vi "3.0-Open FPGA ref and Startup.vi"() -> (0 "queue out":refnum<queue>)   [LabVIEW 2010]
uses:
  2-Low Neurons/2-FPGA VI Typedef.ctl
  2-Low Neurons/2.1-Act Command Typedef.ctl
  2-Low Neurons/2.1 PID Gains Typedef.ctl
  <vilib>/userDefined/High Color/nirio_resource_hc.ctl
  <vilib>/rvi/interface/nirviOpenFPGA/nirviOpenFPGA.xnode
  FPGA Bitfiles/1Hindbrain.lvbitx
  1-Hindbrain.vi
  <vilib>/rvi/ClientSDK/nirviWhatTheDeviceIsDoing.ctl
  <vilib>/rvi/interface/nirviReadWriteControl/nirviReadWriteControl.xnode
  <vilib>/rvi/interface/common/niFpgaNodeNameForErrorReporting.ctl
  <vilib>/rvi/errors/niLvFpgaWhatHappensToTopLevelVI.ctl
  <vilib>/FPGAPlugInAG/cRIO-9104/niLvFpga_Open_cRIO-9104.vi
  <vilib>/Utility/error.llb/Error Cluster From Error Code.vi
  <vilib>/rvi/errors/niLvFpgaAdjustHostInterfaceError.vi
  NiFpgaLv.dll
panel:
  out "error out":errorcluster
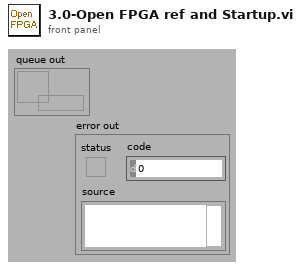
[diagram p1: front panel]
types:
  T1 = typedef "2.1-Act Command Typedef.ctl" = cluster{"Inhibit All Motors":bool, "2.1 Direct Override":bool, "Drive Speed Integer Setpoint":i32, "Steering Integer Setpoint":i32, "Lidar Position Integer Setpoint":i32, "Drive Direct":fxp<+/-,20,5>, "Steer Direct":fxp<+/-,20,5>, "Lidar Direct ":fxp<+/-,20,5>, "2.1.3 Drive PID Gains":T2, "Drive Limit":fxp<+/-,20,5>, "2.1.2 Steering Input C":fxp<+,8,-2>, "2.1.2 Steering Input K":fxp<+/-,14,-6>, "2.1.2 Steering Input F":fxp<+/-,20,5>, "Use NI-9505":bool}
  T2 = typedef "2.1 PID Gains Typedef.ctl" = cluster{"P Gain":fxp<+/-,18,1>, "I Gain":fxp<+/-,18,1>, "D Gain":fxp<+/-,18,1>, "P Gain - Exp":i8, "I Gain - Exp":i8, "D Gain - Exp":i8, "I Saturate":fxp<+/-,64,46>}
  T3 = typedef "2-FPGA VI Typedef.ctl" = refnum<k20>
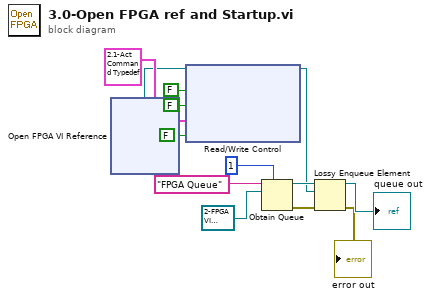
[diagram p0: block diagram]
diagram:
  n1 = xnode "Open FPGA VI Reference"() -> ("FPGA VI Reference Out"=w7:T3)  [unwired: 2 in, 1 out]
  n2 = xnode "Read/Write Control"("FPGA VI Reference In"=w7, "Begin"=FALSE, "Restart"=FALSE, "2.1 Act Command"=T1 {"Inhibit All Motors"=TRUE, "2.1 Direct Override"=TRUE, "Drive Speed Integer Setpoint"=0, "Steering Integer Setpoint"=0, "Lidar Position Integer Setpoint"=0, "Drive Direct"=0.0, "Steer Direct"=0.0, "Lidar Direct "=0.0, "2.1.3 Drive PID Gains"={"P Gain"=0.25, "I Gain"=0.25, "D Gain"=0.25, "P Gain - Exp"=2, "I Gain - Exp"=2, "D Gain - Exp"=2, "I Saturate"=0.25}, "Drive Limit"=0.0, "2.1.2 Steering Input C"=0.0, "2.1.2 Steering Input K"=0.0, "2.1.2 Steering Input F"=0.0, "Use NI-9505"=FALSE}, "stop"=FALSE) -> ("FPGA VI Reference Out"=w5:T3)  [unwired: 1 in, 1 out]
  n3 = Obtain Queue(max queue size (-1, unlimited)=1, name (unnamed)="FPGA Queue", element data type=T3 refnum ("FPGA VI Reference Out")) -> (queue out=w8:refnum<queue>, error out=w9:errorcluster)  [unwired: 2 in, 1 out]
  n4 = Lossy Enqueue Element(queue=w8, element=w5, error in (no error)=w9) -> (queue out=→"queue out":refnum<queue>, error out=→"error out":errorcluster)  [unwired: 2 out]
